vi "Hardware Device Get Info.vi"(8 "error in":errorcluster, 11 "NI Waveform Output in":refnum<class "NI Waveform Output.lvclass">) -> (0 "error out":errorcluster, 3 "NI Waveform Output out":refnum<class "NI Waveform Output.lvclass">)   [LabVIEW 2023, in "HardwareAbstractionLayer_LVOOP.lvlib" / "NI Waveform Output.lvclass"]
doc: "This VI Device Physical Channel Read"
uses:
  NI Waveform Output.lvclass
  NI Waveform Output.lvclass/NI Waveform Output.ctl
  <resource>/objmgr/daqmx.rc
  Teststand/Teststand.lvclass
panel:
  out "AO.WaveformPhysicalChans":tag[](array[tag])
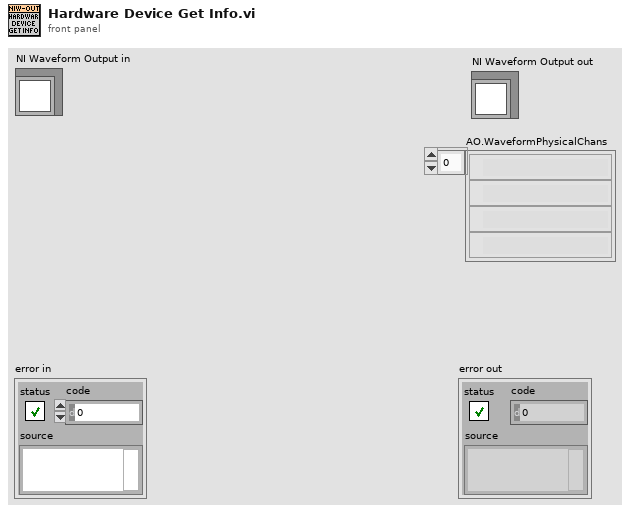
[diagram p1: front panel]
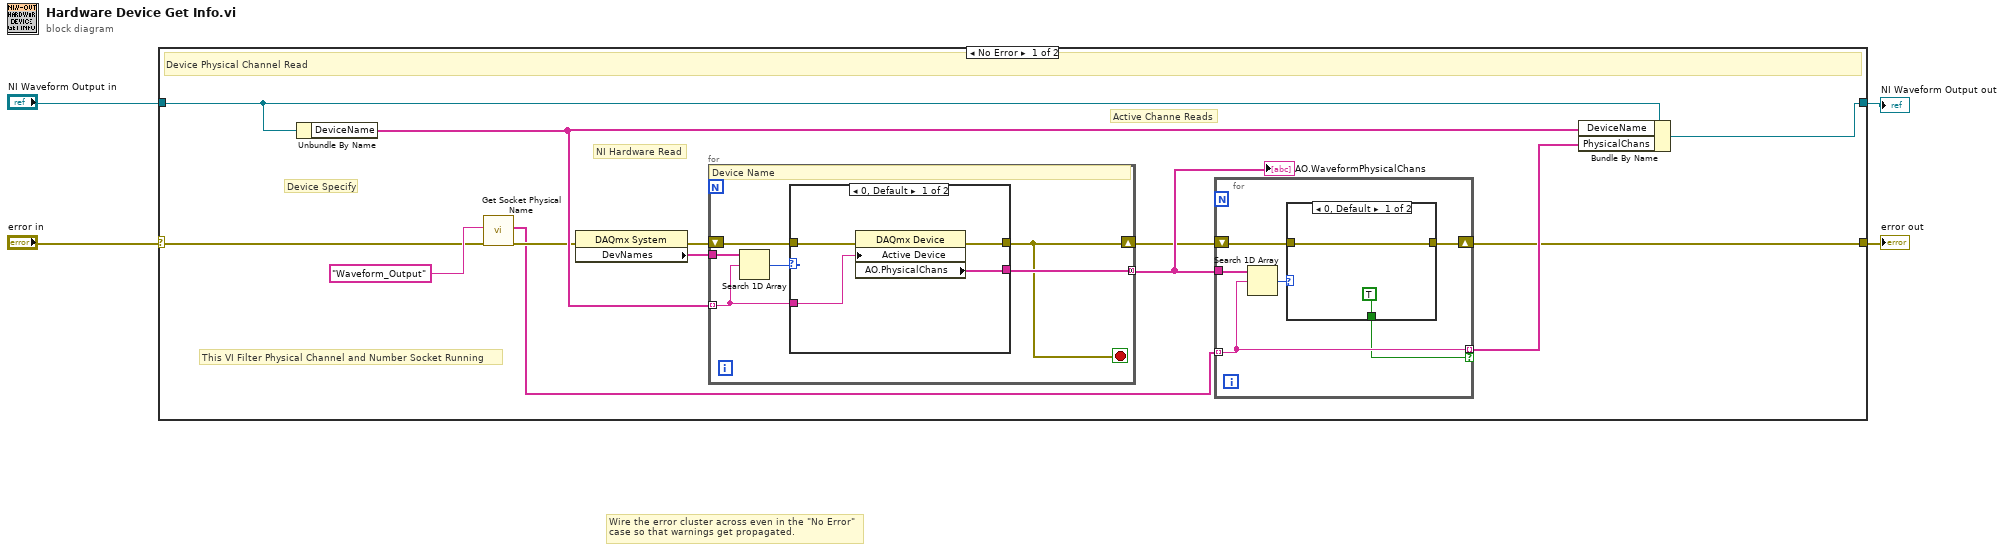
[diagram p0: block diagram]
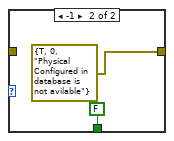
[diagram p2: hidden frame]
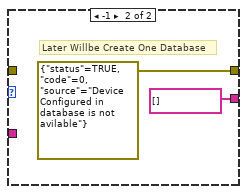
[diagram p3: hidden frame]
diagram:
  # "Wire the error cluster across even in the \"No Error\"\ncase so that warnings get propagated."
  n1 = case shown="No Error" "error in" {
    selector: "error in" -> [w9 w41]
    tunnel: [w7 w41] -> w3
    tunnel: [w6 w40] -> w1
    tunnel: "NI Waveform Output in" -> [w12 w40]
    frame No Error {
      # "This VI Filter Physical Channel and Number Socket Running"
      # "Active Channe Reads"
      # "Device Specify"
      # "NI Hardware Read"
      # "Device Physical Channel Read"
      n2 = Unbundle By Name(w12) -> ("DeviceName"=w17:tag[])
      n3 = call "Get Socket Physical Name.vi"("error In"=w9, "ChannelType"="Waveform_Output") -> ("error out"=w8:errorcluster, "Physical Channel"=w5:tag[])  [unwired: 7 in, 1 out]
      n4 = property class="DAQmx System"(error in=w8) -> (error out=w15:errorcluster, "DevNames"=w16:tag[])  [unwired: 1 in, 1 out]
      n5 = for {
        tunnel: w17 -> [w30] mode=indexing
        tunnel: w16 -> [w31]
        tunnel: [w29] -> w14 mode=concatenating
        shift-right: [w28] -> w13
        shift-left: w15 -> [w32]
        stop <- w28 stop-if-true
        # "Device Name"
        n6 = Search 1D Array(1D array=w31, element=w30) -> (index of element=w33:i32)  [unwired: 1 in]
        n7 = case shown="0, Default" w33 {
          tunnel: w32 -> [w35 _]
          tunnel: [w34 errorcluster {"status"=TRUE, "code"=0, "source"="Device  Configured in database is not avilable"} ("error out")] -> w28
          tunnel: w30 -> [w37 _]
          tunnel: [w36 tag[] [] ("AI.PhysicalChans")] -> w29
          frame 0, Default {
            n8 = property class="DAQmx Device"(error in=w35, "Active Device"=w37) -> (error out=w34:errorcluster, "AO.PhysicalChans"=w36:tag[])  [unwired: 1 in, 1 out]
          }
          frame -1 {
            # "Later Willbe Create One Database"
          }
        }
      }
      "AO.WaveformPhysicalChans" <- w14
      n9 = for {
        tunnel: w14 -> [w23]
        tunnel: w5 -> [w19] mode=indexing
        shift-right: [w20] -> w7
        shift-left: w13 -> [w21]
        tunnel: [w19] -> w11 mode=indexing if=w18
        n10 = Search 1D Array(1D array=w23, element=w19) -> (index of element=w22:i32)  [unwired: 1 in]
        n11 = case shown="0, Default" w22 {
          tunnel: w21 -> [w25 _]
          tunnel: [w25 errorcluster {"status"=TRUE, "code"=0, "source"="Physical Configured in database is not avilable"} ("error out")] -> w20
          tunnel: [TRUE FALSE] -> w18
          frame 0, Default {
          }
          frame -1 {
          }
        }
      }
      n12 = Bundle By Name(cluster=w12, "DeviceName"=w17, "PhysicalChans"=w11) -> (w6:refnum<class "NI Waveform Output.lvclass">)
    }
    frame Error {
    }
  }
  "error out" <- w3
  "NI Waveform Output out" <- w1
